vi "SetLimitExpression.vi"(8 "error in":errorcluster, 10 "LimitExpression":string, 11 "MeasureLimit in":refnum<class "MeasureLimit.lvclass">) -> (0 "error out":errorcluster, 3 "MeasureLimit out":refnum<class "MeasureLimit.lvclass">)   [LabVIEW 2021, in "ProligentXMLGenerator.lvlib" / "MeasureLimit.lvclass"]
doc: "Defines the actual date where the step run ended.\n\nThis value is restricted to \"1900-01-01T00:00:00Z\" -\"2100-01-01T00:00:00Z\"."
uses:
  MeasureLimit.lvclass
  MeasureLimit.lvclass/MeasureLimit.ctl
  Base/NonEmptyString_2000/NonEmptyString_2000.lvclass
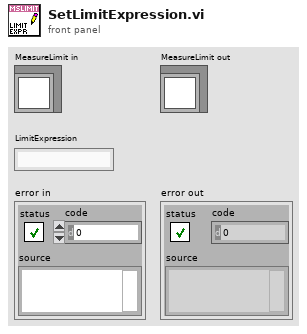
[diagram p1: front panel]
types:
  T1 = typedef "ProligentXMLGenerator.lvlib/MeasureLimit.lvclass/Data.ctl" = cluster{"Name":string, "CustomData":refnum<class "CustomData.lvclass">, "LimitExpression":refnum<class "NonEmptyString_2000.lvclass">}
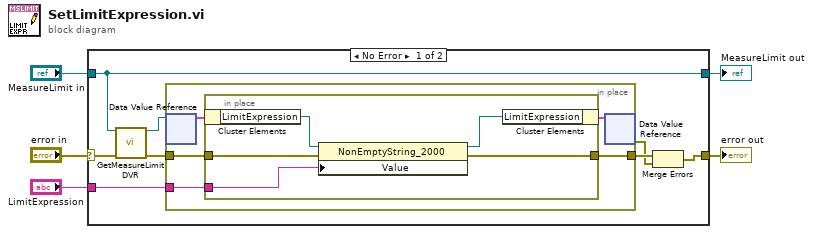
[diagram p0: block diagram]
diagram:
  n1 = case shown="No Error" "error in" {
    selector: "error in" -> [w12 w24]
    tunnel: "MeasureLimit in" -> [w7 w25]
    tunnel: [w9 w24] -> w3
    tunnel: "LimitExpression" -> [w8 _]
    tunnel: [w7 w25] -> w1
    frame No Error {
      n2 = call "GetMeasureLimitDVR.vi"("error in"=w12, "MeasureLimit"=w7) -> ("error out"=w11:errorcluster, "DVRReference"=w13:refnum<data-value>)  [unwired: 8 in]
      n3 = in-place "In Place Element Structure" {
        in-place-border: w11 -> [w16]
        in-place-border: [w18] -> w10
        in-place-border: w8 -> [w17]
        n4 = in-place-dvr #1(w13) -> (w15:T1)  [unwired: 1 out]
        n5 = in-place "In Place Element Structure" {
          in-place-border: [w23] -> w18
          in-place-border: w17 -> [w22]
          in-place-border: w16 -> [w21]
          n6 = in-place-cluster #2(w15) -> ("LimitExpression"=w20:refnum<class "NonEmptyString_2000.lvclass">)
          n7 = property on="Property Node" class="NonEmptyString_2000"(reference=w20, error in=w21, "Value"=w22) -> (reference out=w19:refnum<class "NonEmptyString_2000.lvclass">, error out=w23:errorcluster)
          n8 = in-place-cluster #2("LimitExpression"=w19) -> (w14:T1)
        }
        n9 = in-place-dvr #1(w14) -> (w6:errorcluster)  [unwired: 1 out]
      }
      n10 = Merge Errors(w10, w6) -> (w9:errorcluster)
    }
    frame Error {
    }
  }
  "error out" <- w3
  "MeasureLimit out" <- w1
